vi "controlRobot.vi"(0 "drive":string="drive", 1 "xbox":string="xbox", 3 "shooter":string="shooter", 8 "xbox1":string="xbox1", 9 "gear":string="gear", 10 "shooter":string="shooter", 11 "intake":string="intake") -> ()   [LabVIEW 2016]
uses:
  <vilib>/Rock Robotics/WPI/Utilities/WPI_GetSetVariantRefNum.vi
  2ndContollerStatus.vi
  External.lvlib
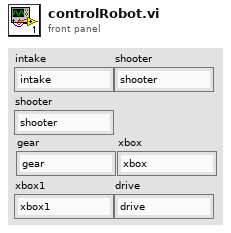
[diagram p1: front panel]
types:
  T1 = typedef "WPI_JoystickDevRef.ctl" = cluster{"Device":T2}
  T2 = typedef "WPI_JoystickDeviceEnum.ctl" = enum16{"USB 0", "USB 1", "USB 2", "USB 3", "USB 4", "USB 5"}
  T3 = typedef "WPI_RobotDriveDevRef.ctl" = cluster{"DevStatus":errorcluster, "Motors[]":T4[], "Square Inputs":bool, "Max Output":dbl}
  T4 = typedef "WPI_MotorControlDeviceRef.ctl" = cluster{"DeviceStatus":errorcluster, "Type":T5, "PWM":cluster{"PWM Channel":T6, "DeadBand":T7}, "CAN":cluster{"Device Number":u8, "SetOutput VI Ref":variant, "GetOutput VI Ref":variant, "Enable VI Ref":variant, "Disable VI Ref":variant, "Data":variant}, "Invert":bool}
  T5 = typedef "WPI_MotorControlType.ctl" = enum16{"PWM", "CAN"}
  T6 = typedef "FPGA_DIOPWMChannel.ctl" = enum8{"PWM 0", "PWM 1", "PWM 2", "PWM 3", "PWM 4", "PWM 5", "PWM 6", "PWM 7", "PWM 8", "PWM 9", "PWM MXP 0", "PWM MXP 1", "PWM MXP 2", "PWM MXP 3", "PWM MXP 4", "PWM MXP 5", "PWM MXP 6", "PWM MXP 7", "PWM MXP 8", "PWM MXP 9", "Invalid"}
  T7 = typedef "WPI_PWMDeadband.ctl" = cluster{"Name":string, "maxPositivePwm":i32, "minPositivePwm":i32, "centerPwm":i32, "maxNegativePwm":i32, "minNegativePwm":i32, "angularRange":u16}
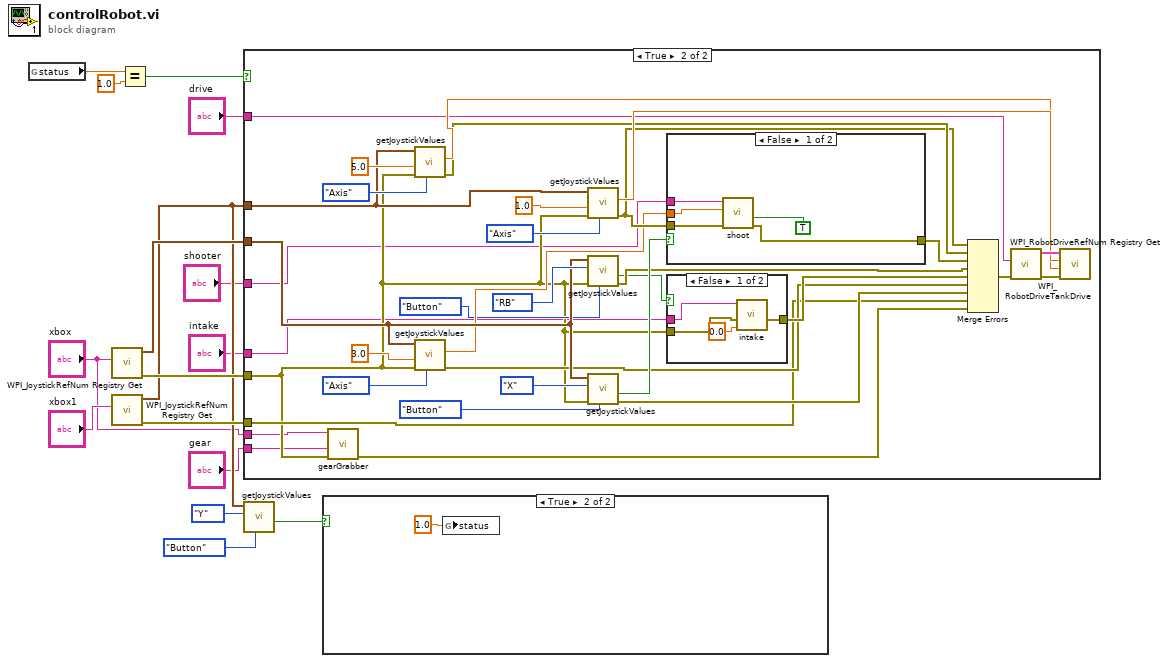
[diagram p0: block diagram]
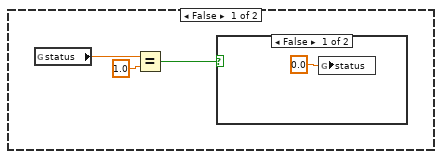
[diagram p2: hidden frame]
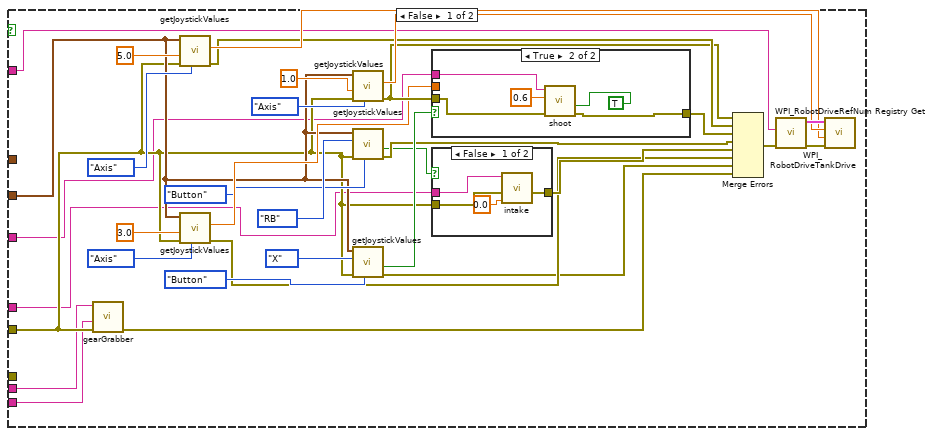
[diagram p4: hidden frame]
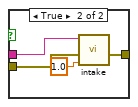
[diagram p5: hidden frame]
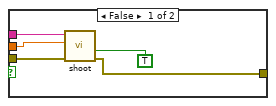
[diagram p6: hidden frame]
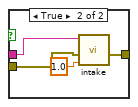
[diagram p7: hidden frame]
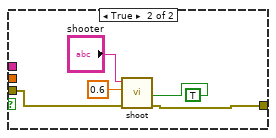
[diagram p8: hidden frame]
diagram:
  n1 = global read "2ndContollerStatus.vi" "status"() -> (w8:dbl)
  n2 = call <vilib>:"WPI_JoystickRefNum Registry Get.vi"("refnum name"="xbox") -> ("error out"=w15:errorcluster, "JoystickDevRef"=w16:T1)  [unwired: 9 in]
  n3 = call <vilib>:"WPI_JoystickRefNum Registry Get.vi"("refnum name"="xbox1") -> ("error out"=w13:errorcluster, "JoystickDevRef"=w12:T1)  [unwired: 9 in]
  n4 = Equal?(x=w8, y=1.0) -> (x = y?=w6:bool)
  n5 = case shown="True" w6 {
    tunnel: w16 -> [w25 w84]
    tunnel: w15 -> [w24 w75]
    tunnel: w12 -> [_ w77]
    tunnel: w13 -> [_ w76]
    tunnel: "xbox" -> [w21 w72]
    tunnel: "gear" -> [w20 w71]
    tunnel: "intake" -> [w18 w70]
    tunnel: "shooter" -> [w19 w69]
    tunnel: "drive" -> [w17 w68]
    frame False {
      n6 = call "gearGrabber.vi"("error in (no error)"=w24, "gear"=w20, "xbox"=w21) -> ("error out"=w22:errorcluster)  [unwired: 8 in]
      n7 = call "getJoystickValues.vi"("Mode"=enum16{"Axis", "Button"}."Axis", "error in (no error)"=w24, "Axis"=5.0, "JoystickDevRef"=w25) -> ("error out"=w41:errorcluster, "Value"=w44:dbl)  [unwired: 4 in, 2 out]
      n8 = call "getJoystickValues.vi"("Mode"=enum16{"Axis", "Button"}."Axis", "error in (no error)"=w24, "Axis"=3.0, "JoystickDevRef"=w25) -> ("error out"=w30:errorcluster, "Value"=w27:dbl)  [unwired: 4 in, 2 out]
      n9 = call "getJoystickValues.vi"("Mode"=enum16{"Axis", "Button"}."Axis", "error in (no error)"=w24, "Axis"=1.0, "JoystickDevRef"=w25) -> ("error out"=w39:errorcluster, "Value"=w45:dbl)  [unwired: 4 in, 2 out]
      n10 = call "getJoystickValues.vi"("Mode"=enum16{"Axis", "Button"}."Button", "error in (no error)"=w24, "buttonType"=enum16{"A", "B", "X", "Y", "LB", "RB"}."RB", "JoystickDevRef"=w25) -> ("error out"=w35:errorcluster, "Button Pressed"=w32:bool)  [unwired: 4 in, 2 out]
      n11 = call "getJoystickValues.vi"("Mode"=enum16{"Axis", "Button"}."Button", "error in (no error)"=w24, "buttonType"=enum16{"A", "B", "X", "Y", "LB", "RB"}."X", "JoystickDevRef"=w25) -> ("error out"=w28:errorcluster, "Button Pressed"=w42:bool)  [unwired: 4 in, 2 out]
      n12 = case shown="True" w42 {
        tunnel: w39 -> [w62 w67]
        tunnel: [w61 w66] -> w38
        tunnel: w27 -> [w59 _]
        tunnel: w19 -> [w58 w63]
        frame False {
          n13 = call "shoot.vi"("Shooting Activated"=TRUE, "error in (no error)"=w62, "Motor Power"=w59, "refnum name"=w58) -> ("error out"=w61:errorcluster)  [unwired: 7 in]
        }
        frame True {
          n14 = call "shoot.vi"("Shooting Activated"=TRUE, "error in (no error)"=w67, "Motor Power"=0.6, "refnum name"=w63) -> ("error out"=w66:errorcluster)  [unwired: 7 in]
        }
      }
      n15 = case shown="False" w32 {
        tunnel: w24 -> [w52 w57]
        tunnel: [w51 w56] -> w34
        tunnel: w18 -> [w50 w54]
        frame False {
          n16 = call "intake.vi"("intakeSpeed"=0.0 ("intake speed"), "error in (no error)"=w52, "intake"=w50) -> ("error out"=w51:errorcluster)  [unwired: 8 in]
        }
        frame True {
          n17 = call "intake.vi"("intakeSpeed"=1.0 ("intake speed"), "error in (no error)"=w57, "intake"=w54) -> ("error out"=w56:errorcluster)  [unwired: 8 in]
        }
      }
      n18 = Merge Errors(w39, w41, w38, w35, w34, w30, w28, w22) -> (w23:errorcluster)
      n19 = call <vilib>:"WPI_RobotDriveRefNum Registry Get.vi"("error in (no error)"=w23, "refnum name"=w17) -> ("error out"=w48:errorcluster, "RobotDriveDevRef"=w49:T3)  [unwired: 8 in]
      n20 = call <vilib>:"WPI_RobotDriveTankDrive.vi"("error in (no error)"=w48, "Right axis value"=w44, "Left axis value"=w45, "RobotDriveDevRef"=w49) -> ()  [unwired: 5 in, 3 out]
    }
    frame True {
      n21 = call "gearGrabber.vi"("error in (no error)"=w75, "gear"=w71, "xbox"=w72) -> ("error out"=w74:errorcluster)  [unwired: 8 in]
      n22 = call "getJoystickValues.vi"("Mode"=enum16{"Axis", "Button"}."Axis", "error in (no error)"=w75, "Axis"=5.0, "JoystickDevRef"=w77) -> ("error out"=w94:errorcluster, "Value"=w97:dbl)  [unwired: 4 in, 2 out]
      n23 = call "getJoystickValues.vi"("Mode"=enum16{"Axis", "Button"}."Axis", "error in (no error)"=w75, "Axis"=3.0, "JoystickDevRef"=w84) -> ("error out"=w82:errorcluster, "Value"=w79:dbl)  [unwired: 4 in, 2 out]
      n24 = call "getJoystickValues.vi"("Mode"=enum16{"Axis", "Button"}."Axis", "error in (no error)"=w75, "Axis"=1.0, "JoystickDevRef"=w77) -> ("error out"=w92:errorcluster, "Value"=w98:dbl)  [unwired: 4 in, 2 out]
      n25 = call "getJoystickValues.vi"("Mode"=enum16{"Axis", "Button"}."Button", "error in (no error)"=w75, "buttonType"=enum16{"A", "B", "X", "Y", "LB", "RB"}."RB", "JoystickDevRef"=w84) -> ("error out"=w88:errorcluster, "Button Pressed"=w85:bool)  [unwired: 4 in, 2 out]
      n26 = call "getJoystickValues.vi"("Mode"=enum16{"Axis", "Button"}."Button", "error in (no error)"=w75, "buttonType"=enum16{"A", "B", "X", "Y", "LB", "RB"}."X", "JoystickDevRef"=w84) -> ("error out"=w80:errorcluster, "Button Pressed"=w95:bool)  [unwired: 4 in, 2 out]
      n27 = case shown="False" w95 {
        tunnel: w92 -> [w115 w119]
        tunnel: [w114 w118] -> w91
        tunnel: w79 -> [w112 _]
        tunnel: w69 -> [w111 _]
        frame False {
          n28 = call "shoot.vi"("Shooting Activated"=TRUE, "error in (no error)"=w115, "Motor Power"=w112, "refnum name"=w111) -> ("error out"=w114:errorcluster)  [unwired: 7 in]
        }
        frame True {
          n29 = call "shoot.vi"("Shooting Activated"=TRUE, "error in (no error)"=w119, "Motor Power"=0.6, "refnum name"="shooter") -> ("error out"=w118:errorcluster)  [unwired: 7 in]
        }
      }
      n30 = case shown="False" w85 {
        tunnel: w75 -> [w105 w110]
        tunnel: [w104 w109] -> w87
        tunnel: w70 -> [w103 w107]
        frame False {
          n31 = call "intake.vi"("intakeSpeed"=0.0 ("intake speed"), "error in (no error)"=w105, "intake"=w103) -> ("error out"=w104:errorcluster)  [unwired: 8 in]
        }
        frame True {
          n32 = call "intake.vi"("intakeSpeed"=1.0 ("intake speed"), "error in (no error)"=w110, "intake"=w107) -> ("error out"=w109:errorcluster)  [unwired: 8 in]
        }
      }
      n33 = Merge Errors(w92, w94, w91, w88, w87, w82, w80, w76, w74) -> (w73:errorcluster)
      n34 = call <vilib>:"WPI_RobotDriveRefNum Registry Get.vi"("error in (no error)"=w73, "refnum name"=w68) -> ("error out"=w101:errorcluster, "RobotDriveDevRef"=w102:T3)  [unwired: 8 in]
      n35 = call <vilib>:"WPI_RobotDriveTankDrive.vi"("error in (no error)"=w101, "Right axis value"=w97, "Left axis value"=w98, "RobotDriveDevRef"=w102) -> ()  [unwired: 5 in, 3 out]
    }
  }
  n36 = call "getJoystickValues.vi"("Mode"=enum16{"Axis", "Button"}."Button", "buttonType"=enum16{"A", "B", "X", "Y", "LB", "RB"}."Y", "JoystickDevRef"=w12) -> ("Button Pressed"=w9:bool)  [unwired: 5 in, 3 out]
  n37 = case shown="True" w9 {
    frame False {
      n38 = global read "2ndContollerStatus.vi" "status"() -> (w123:dbl)
      n39 = Equal?(x=w123, y=1.0) -> (x = y?=w121:bool)
      n40 = case shown="False" w121 {
        frame False {
          n41 = global write "2ndContollerStatus.vi" "status"(0.0 ("status")) -> ()
        }
        frame True {
        }
      }
    }
    frame True {
      n42 = global write "2ndContollerStatus.vi" "status"(1.0 ("status")) -> ()
    }
  }
